vi "AutoSubroutine.vi"(8 "error in (no error)":errorcluster, 11 "AutoSubsystem in":refnum<class "AutoSubroutine.lvclass">) -> (0 "error out":errorcluster, 3 "AutoSubsystem out":refnum<class "AutoSubroutine.lvclass">)   [LabVIEW 2017, in "AutoSubroutine.lvclass"]
uses:
  AutoSubroutine.lvclass
  AutoSubroutine.lvclass/AutoSubroutine.ctl
  Subsystem/Subsystem.lvclass
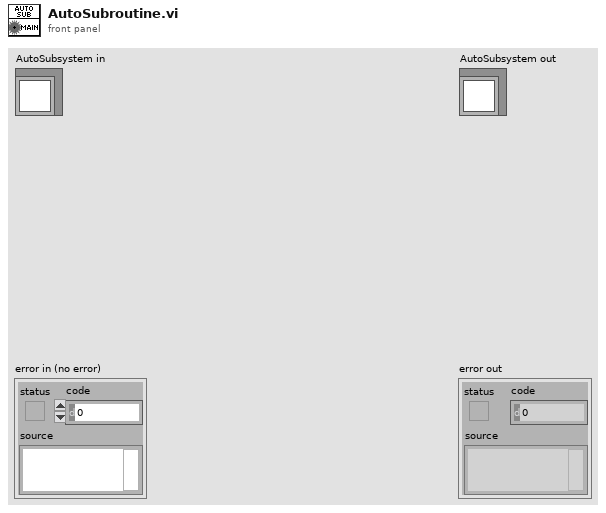
[diagram p1: front panel]
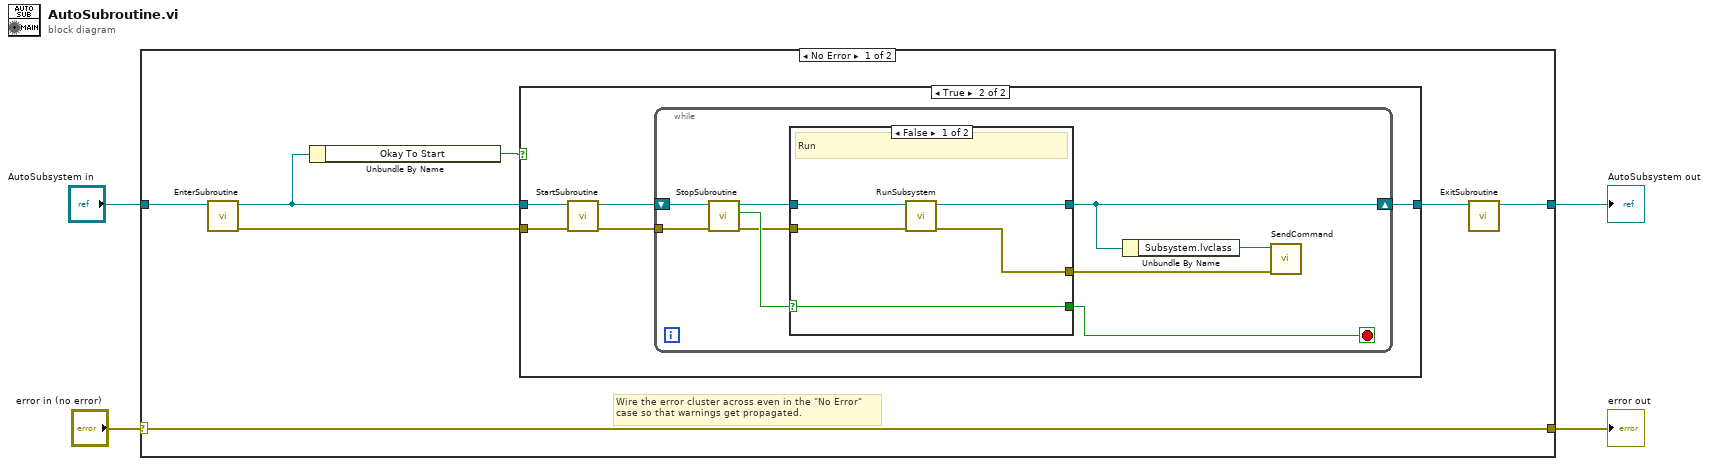
[diagram p0: block diagram]
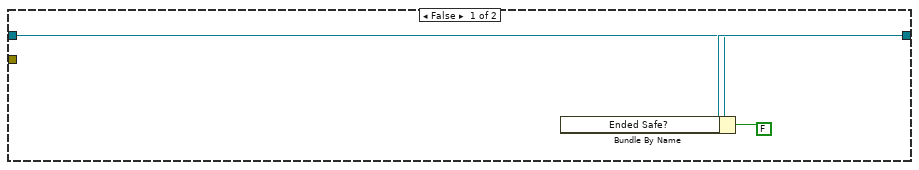
[diagram p2: hidden frame]
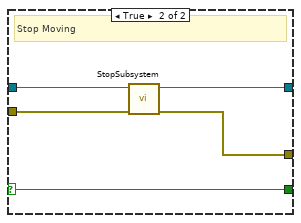
[diagram p3: hidden frame]
diagram:
  n1 = case shown="No Error" "error in (no error)" {
    selector: "error in (no error)" -> [w11 w40]
    tunnel: [w11 w40] -> w3
    tunnel: [w6 w39] -> w1
    tunnel: "AutoSubsystem in" -> [w10 w39]
    frame No Error {
      # "Wire the error cluster across even in the \"No Error\"\ncase so that warnings get propagated."
      n2 = call-dynamic "EnterSubroutine.vi"("AutoSubroutine in"=w10) -> ("error out"=w5:errorcluster, "AutoSubroutine out"=w9:refnum<class "AutoSubroutine.lvclass">)  [unwired: 9 in]
      n3 = Unbundle By Name(w9) -> ("Okay To Start"=w8:bool)
      n4 = case shown="True" w8 {
        tunnel: w9 -> [w13 w18]
        tunnel: [w14 w19] -> w7
        tunnel: w5 -> [_ w16]
        frame False {
          n5 = Bundle By Name(cluster=w13, "Ended Safe?"=FALSE ("AutoGeneralOut.Ended Safe?")) -> (w14:refnum<class "AutoSubroutine.lvclass">)
        }
        frame True {
          n6 = call-dynamic "StartSubroutine.vi"("error in (no error)"=w16, "AutoSubroutine in"=w18) -> ("error out"=w15:errorcluster, "AutoSubroutine out"=w17:refnum<class "AutoSubroutine.lvclass">)  [unwired: 8 in]
          n7 = while {
            shift-right: [w24] -> w19
            shift-left: w17 -> [w28]
            tunnel: w15 -> [w22]
            stop <- w25 stop-if-true
            n8 = call-dynamic "StopSubroutine.vi"("error in (no error)"=w22, "AutoSubroutine in"=w28) -> ("error out"=w21:errorcluster, "Stop Loop?"=w26:bool, "AutoSubroutine out"=w27:refnum<class "AutoSubroutine.lvclass">)  [unwired: 7 in]
            n9 = case shown="False" w26 {
              selector: w26 -> [w33 w38]
              tunnel: [w31 w36] -> w24
              tunnel: w27 -> [w32 w37]
              tunnel: [w33 w38] -> w25
              tunnel: w21 -> [w30 w35]
              tunnel: [w29 w34] -> w20
              frame False {
                # "Run"
                n10 = call-dynamic "RunSubsystem.vi"("error in (no error)"=w30, "AutoSubroutine in"=w32) -> ("error out"=w29:errorcluster, "AutoSubroutine out"=w31:refnum<class "AutoSubroutine.lvclass">)  [unwired: 8 in]
              }
              frame True {
                # "Stop Moving"
                n11 = call-dynamic "StopSubsystem.vi"("error in (no error)"=w35, "AutoSubroutine in"=w37) -> ("error out"=w34:errorcluster, "AutoSubroutine out"=w36:refnum<class "AutoSubroutine.lvclass">)  [unwired: 8 in]
              }
            }
            n12 = Unbundle By Name(w24) -> ("Subsystem.lvclass"=w23:refnum<class "Subsystem.lvclass">)
            n13 = call-dynamic "SendCommand.vi"("error in (no error)"=w20, "Subsystem in"=w23) -> ()  [unwired: 7 in, 3 out]
          }
        }
      }
      n14 = call-dynamic "ExitSubroutine.vi"("AutoSubroutine in"=w7) -> ("AutoSubroutine out"=w6:refnum<class "AutoSubroutine.lvclass">)  [unwired: 9 in, 1 out]
    }
    frame Error {
    }
  }
  "error out" <- w3
  "AutoSubsystem out" <- w1
